vi "SQL_Update.vi"(6 "查询语句":string, 7 "表名":string, 8 "error in (no error)":errorcluster, 9 "列名对应的值":string[](array[string]), 10 "列名":string[](array[string]), 11 "connection reference":T1) -> (0 "error out":errorcluster, 3 "connection reference 2":T1)   [LabVIEW 2018]
uses:
  <vilib>/addons/database/Connection.llb/Conn ObjectReference.ctl
  <vilib>/addons/database/Connection.llb/Conn Execute.vi
  <vilib>/addons/database/Recordset.llb/Rec Destroy - Connection.vi
  <vilib>/addons/database/NI_Database_API.lvlib
panel:
  # "语法："
  # "UPDATE 表名称 SET 列名称 = 新值 WHERE 列名称 = 某值"
  # "例：where a='1'"
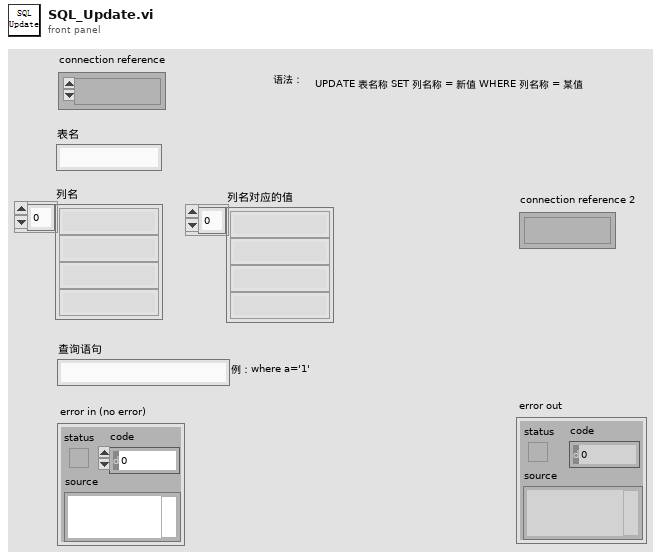
[diagram p1: front panel]
types:
  T1 = typedef "NI_Database_API.lvlib/Conn ObjectReference.ctl" = refnum<k1>
  T2 = typedef "NI_Database_API.lvlib/Rec ObjectReference.ctl" = refnum<k1>
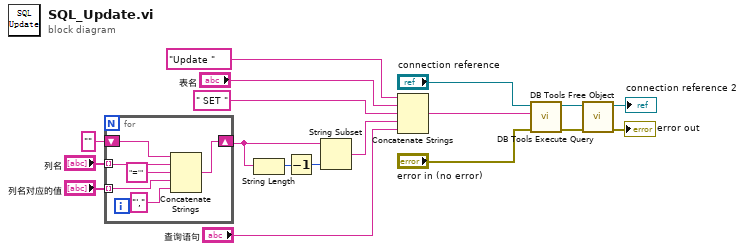
[diagram p0: block diagram]
diagram:
  n1 = for {
    tunnel: "列名" -> [w24] mode=indexing
    tunnel: "列名对应的值" -> [w22] mode=indexing
    shift-right: [w20] -> w8
    shift-left: "" -> [w19]
    n2 = Concatenate Strings(w19, w24, "='" ("字符串"), w22, "'," ("字符串")) -> (w20:string)
  }
  n3 = String Length(string=w8) -> (length=w6:i32)
  n4 = Decrement(x=w6) -> (x-1=w7:i32)
  n5 = String Subset(string=w8, length (rest)=w7) -> (substring=w5:string)  [unwired: 1 in]
  n6 = Concatenate Strings("Update ", "表名", " SET " ("字符串"), w5, "查询语句") -> (w16:string)
  n7 = call-poly <vilib>:"DB Tools Execute Query.vi"("error in (no error)"="error in (no error)", "SQL query"=w16, "connection reference"="connection reference") -> ("error out"=w2:errorcluster, "recordset reference"=w3:T2)  [unwired: 5 in]
  n8 = call-poly <vilib>:"DB Tools Free Object.vi"("error in (no error)"=w2, "recordset reference"=w3) -> ("error out"=→"error out":errorcluster, "connection reference"=→"connection reference 2":T1)  [unwired: 8 in]
